vi "Send_Command.vi"(8 "error in (no error)":errorcluster, 10 "write buffer":string, 11 "Serial Port in":refnum<visa-resource-name>) -> (0 "error out":errorcluster, 2 "Read buffer":string, 3 "VISA Refnum out":refnum<visa-resource-name>)   [LabVIEW 2016, in "Chemyx_Syringe_Pump_driver.lvlib"]
uses:
  Chemyx_Syringe_Pump_driver.lvlib
panel:
  # "Returns the elapsed time of the current operation of the pump as a number of seconds and as a string formatted as X hr YY min ZZ sec."
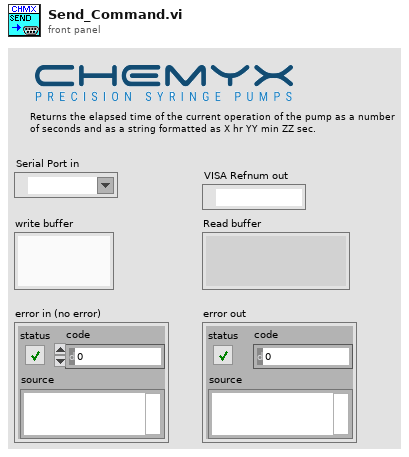
[diagram p1: front panel]
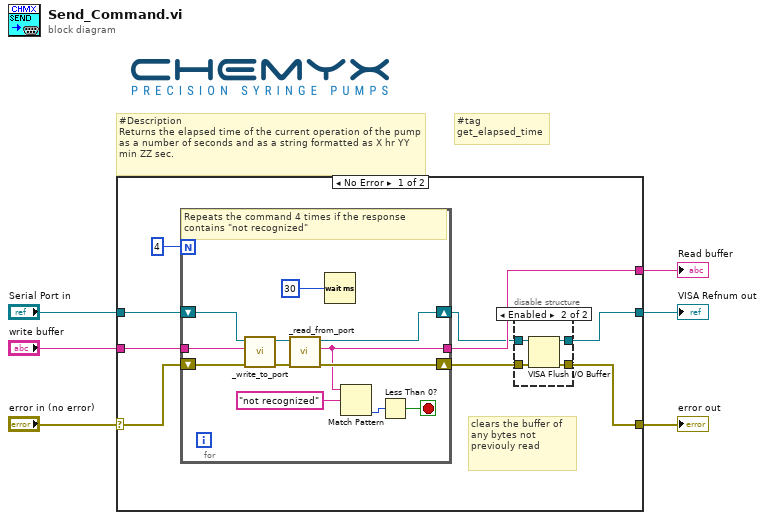
[diagram p0: block diagram]
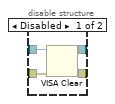
[diagram p2: hidden frame]
diagram:
  # "#tag\nget_elapsed_time"
  # "#Description\nReturns the elapsed time of the current operation of the pump as a number of seconds and as a string formatted as X hr YY min ZZ sec."
  n1 = case shown="No Error" "error in (no error)" {
    selector: "error in (no error)" -> [w12 w38]
    tunnel: [w14 w37] -> w6
    tunnel: "write buffer" -> [w13 w37]
    tunnel: "Serial Port in" -> [w11 w36]
    tunnel: [w9 w38] -> w2
    tunnel: [w7 w36] -> w1
    frame No Error {
      # "clears the buffer of any bytes not previouly read"
      n2 = for {
        N: 4 -> [_]
        tunnel: [w28] -> w14
        tunnel: w13 -> [w31]
        shift-right: [w32] -> w15
        shift-left: w12 -> [w30]
        shift-right: [w33] -> w8
        shift-left: w11 -> [w29]
        stop <- w25 stop-if-true
        # "Repeats the command 4 times if the response contains \"not recognized\""
        n3 = call "_write_to_port.vi"("error in (no error)"=w30, "write buffer"=w31, "Serial Port in"=w29) -> ("error out"=w35:errorcluster, "Serial Port out"=w34:refnum<visa-resource-name>)  [unwired: 7 in]
        n4 = call "_read_from_port.vi"("Serial port in"=w34, "error in (no error)"=w35) -> ("Serial port out"=w33:refnum<visa-resource-name>, "Read buffer"=w28:string, "error out"=w32:errorcluster)  [unwired: 5 in, 1 out]
        n5 = Wait (ms)(milliseconds to wait=u32 30) -> ()  [unwired: 1 out]
        n6 = Match Pattern(string=w28, regular expression="not recognized") -> (offset past match=w26:i32)  [unwired: 1 in, 3 out]
        n7 = Less Than 0?(x=w26) -> (x < 0?=w25:bool)
      }
      n8 = disable-structure shown="Enabled" {
        disable-tunnel: w15 -> [w19 w20]
        disable-tunnel: [w18 w21] -> w9
        disable-tunnel: w8 -> [w17 w23]
        disable-tunnel: [w16 w22] -> w7
        frame Disabled {
          n9 = VISA Clear(VISA resource name=w17, error in (no error)=w19) -> (VISA resource name out=w16:refnum<visa-resource-name>, error out=w18:errorcluster)
        }
        frame Enabled {
          n10 = VISA Flush I/O Buffer(VISA resource name=w23, error in (no error)=w20) -> (VISA resource name out=w22:refnum<visa-resource-name>, error out=w21:errorcluster)  [unwired: 1 in]
        }
      }
    }
    frame Error {
    }
  }
  "VISA Refnum out" <- w1
  "error out" <- w2
  "Read buffer" <- w6
